vi "Thev-Plot Data.vi"(0 "Optim":T1, 2 "State":T2={"next"=-1, "ER10X"=refnum, "phase"=enum."Optimize", "progress"=[], "folder"=path "", "log"="", "history"={"L"=[], "F"=[]}, "optim"={"MSE"=0.0, "Niter"=0, "Linit"=[], "Lfinal"=[]}}, 5 "Mag graph":refnum<vi>, 7 "Phase graph":refnum<vi>, 11 "error in (no error)":errorcluster) -> (15 "error out":errorcluster)   [LabVIEW 2015]
doc: "This helper VI loads calibration data from a file, and plots the magnitude and phase on graphs whose references are inputs to the VI. Handles the logic of overplotting data, selecting the colors and linestyles, and inserting the filename into the legend.\n\nKEH 9/10/09"
uses:
  Typedefs/Thev-State.ctl
  D:/Experiment VIs/Misc VIs/Equipment Control/ER10X/ER10XConnect.NET.dll
  Misc VIs/Equipment Control/ER10X/ER10XConnect.NET.dll
  Typedefs/Thev-Procedure Phase.ctl
  Typedefs/Thev-Progress Table Element.ctl
  Typedefs/Thev-Optimization Result.ctl
  Typedefs/Thev-Optimization Parameters.ctl
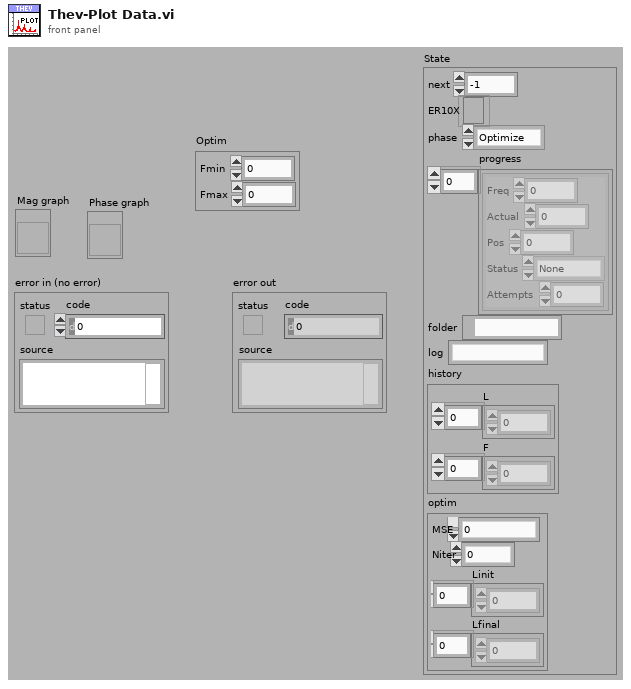
[diagram p1: front panel]
types:
  T1 = typedef "Thev-Optimization Parameters.ctl" = cluster{"Fmin":dbl, "Fmax":dbl}
  T2 = typedef "Thev-State.ctl" = cluster{"next":i32, "ER10X":refnum<k24>, "phase":T3, "progress":T4[], "folder":path, "log":string, "history":cluster{"L":dbl[], "F":dbl[]}, "optim":T5}
  T3 = typedef "Thev-Procedure Phase.ctl" = enum16{"Optimize", "Measure", "Compute", "Finished"}
  T4 = typedef "Thev-Progress Table Element.ctl" = cluster{"Freq":dbl, "Actual":dbl, "Pos":dbl, "Status":enum16{"None", "Measuring", "Finished"}, "Attempts":i32}
  T5 = typedef "Thev-Optimization Result.ctl" = cluster{"MSE":dbl, "Niter":i32, "Linit":dbl[], "Lfinal":dbl[]}
  T6 = enum16{"User", "Prism", "Kelly", "Dark2", "Sequential", "Hue"}
  T7 = cluster{"Frequency (Hz)":dbl[], "Phase (cycles)":dbl[]}
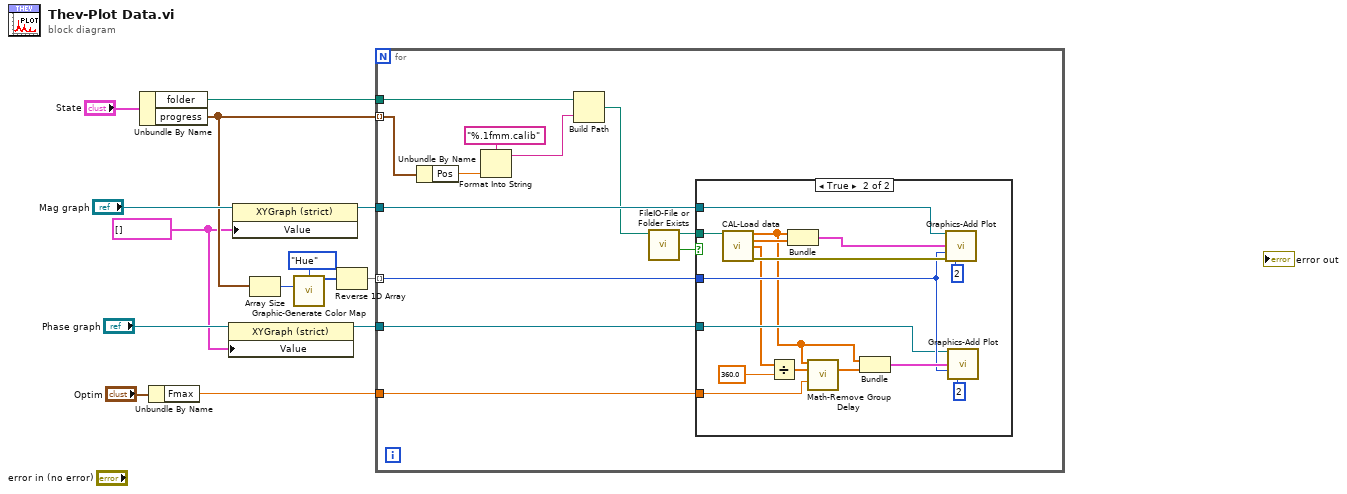
[diagram p0: block diagram]
diagram:
  w3 = cluster{"PTC Mag":dbl[], "PTC Phase":dbl[]}[] [] ("Value")
  n1 = Unbundle By Name("State") -> ("folder"=w12:path, "progress"=w8:T4[])
  n2 = Unbundle By Name("Optim") -> ("Fmax"=w1:dbl)
  n3 = property class="XYGraph (strict)"(reference="Phase graph", "Value"=w3) -> (reference out=w4:refnum<vi>)  [unwired: 1 in, 1 out]
  n4 = property class="XYGraph (strict)"(reference="Mag graph", "Value"=w3) -> (reference out=w6:refnum<vi>)  [unwired: 1 in, 1 out]
  n5 = Array Size(array=w8) -> (size(s)=w9:i32)
  n6 = call "Graphic-Generate Color Map.vi"("Map"=T6."Hue", "Size"=w9) -> ("Colors"=w10:u32[])  [unwired: 13 in]
  n7 = Reverse 1D Array(array=w10) -> (reversed array=w7:u32[])
  n8 = for {
    tunnel: w6 -> [w26]
    tunnel: w12 -> [w21]
    tunnel: w8 -> [w25] mode=indexing
    tunnel: w7 -> [w20] mode=indexing
    tunnel: w4 -> [w16]
    tunnel: w1 -> [w15]
    n9 = Unbundle By Name(w25) -> ("Pos"=w23:dbl)
    n10 = Format Into String(format string="%.1fmm.calib", w23) -> (resulting string=w22:string)  [unwired: 2 in, 1 out]
    n11 = Build Path(base path=w21, name or relative path=w22) -> (appended path=w19:path)
    n12 = call "FileIO-File or Folder Exists.vi"("path"=w19) -> ("Exists?"=w17:bool, "dup path"=w18:path)  [unwired: 7 in, 2 out]
    n13 = case shown="True" w17 {
      tunnel: w26 -> [_ w42]
      tunnel: w20 -> [_ w33]
      tunnel: w18 -> [_ w38]
      tunnel: w16 -> [_ w32]
      tunnel: w15 -> [_ w27]
      frame False {
      }
      frame True {
        n14 = call "CAL-Load data.vi"("user path"=w38) -> ("Frequency (Hz)"=w29:dbl[], "Mag"=w36:dbl[], "Phase"=w31:dbl[], "error out"=w41:errorcluster)  [unwired: 7 in, 4 out]
        n15 = Divide(x=w31, y=360.0) -> (x/y=w30:dbl[])
        n16 = Bundle("Frequency (Hz)"=w29, "Mag"=w36) -> (w40:cluster{"Frequency (Hz)":dbl[], "Mag":dbl[]})  [unwired: 1 in]
        n17 = call "Math-Remove Group Delay.vi"("Frequency (Hz)"=w29, "Phase (cycles)"=w30, "Fmax (Hz)"=w27) -> ("Phase (cycles)"=w28:dbl[])  [unwired: 11 in, 1 out]
        n18 = Bundle("Frequency (Hz)"=w29, "Phase (cycles)"=w28) -> (w34:T7)  [unwired: 1 in]
        n19 = call "Graphics-Add Plot.vi"("XYGraph in"=w42, "XY Data"=w40, "Color"=w33, "error in (no error)"=w41, "Plot.Line Width"=u8 2) -> ()  [unwired: 9 in, 2 out]
        n20 = call "Graphics-Add Plot.vi"("XYGraph in"=w32, "XY Data"=w34, "Color"=w33, "Plot.Line Width"=u8 2) -> ()  [unwired: 10 in, 2 out]
      }
    }
  }
